vi "(SubVI)File Gen_Get Default Path.vi"(8 "error in (no error)":errorcluster caption="에러 입력(에러 없음)", 11 "Common?":bool) -> (0 "error out":errorcluster caption="에러 출력", 3 "default path":path)   [LabVIEW 2020]
uses:
  Variables/(Var)System Variables.vi
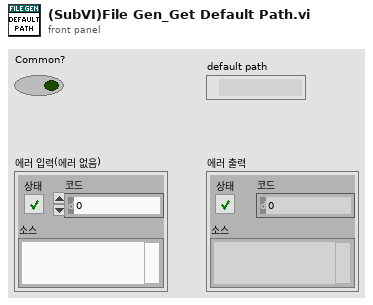
[diagram p1: front panel]
types:
  T1 = typedef "Haptic IC.lvclass/(Ctrl)IC Type.ctl" = enum8{"DW7800", "DW7802", "DW7912", "DW7914"}
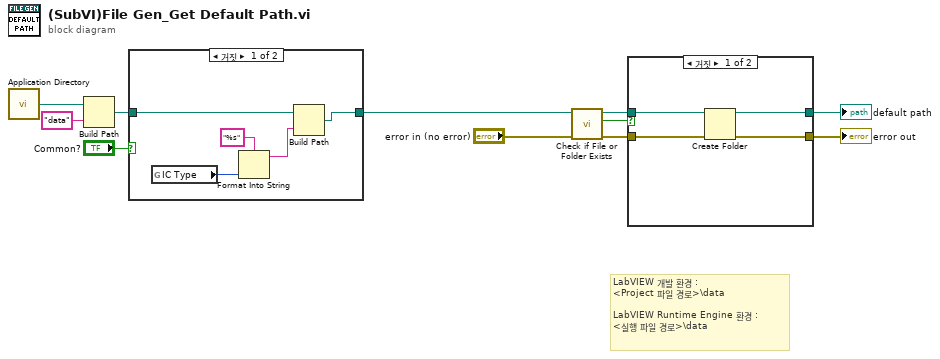
[diagram p0: block diagram]
diagram:
  # "LabVIEW 개발 환경 : \n<Project 파일 경로>\\data\n\nLabVIEW Runtime Engine 환경 : \n<실행 파일 경로>\\data"
  n1 = call <vilib>:"Application Directory.vi"() -> ("Application Directory"=w3:path)
  n2 = Build Path(base path=w3, name or relative path="data") -> (appended path=w2:path)
  n3 = case shown="거짓" "Common?" {
    tunnel: w2 -> [w14 w17]
    tunnel: [w12 w17] -> w1
    frame False {
      n4 = global read "(Var)System Variables.vi" "IC Type"() -> (w16:T1)
      n5 = Format Into String(format string="%s" ("포맷 문자열"), w16) -> (resulting string=w13:string)  [unwired: 2 in, 1 out]
      n6 = Build Path(base path=w14, name or relative path=w13) -> (appended path=w12:path)
    }
    frame True {
    }
  }
  n7 = call <vilib>:"Check if File or Folder Exists.vi"("error in (no error)"="error in (no error)", "path"=w1) -> ("error out"=w9:errorcluster, "file or folder exists?"=w11:bool, "dup path"=w10:path)  [unwired: 7 in]
  n8 = case shown="거짓" w11 {
    tunnel: w10 -> [w19 w23]
    tunnel: [w18 w23] -> w6
    tunnel: w9 -> [w21 w22]
    tunnel: [w20 w22] -> w7
    frame False {
      n9 = Create Folder(path (use dialog)=w19, error in=w21) -> (created path=w18:path, error out=w20:errorcluster)  [unwired: 1 in, 1 out]
    }
    frame True {
    }
  }
  "error out" <- w7
  "default path" <- w6
